vi "Read_VN200.vi"(0 "FPGA Interface":refnum<k20>, 5 "error in":errorcluster) -> (4 "FPGA Interface Out":refnum<k20>, 6 "error out":errorcluster, 8 "Position Data":T1)   [LabVIEW 2016]
uses:
  Typedef/INS Data.ctl
  <vilib>/Utility/error.llb/Error Cluster From Error Code.vi
  <vilib>/rvi/errors/niLvFpgaAdjustHostInterfaceError.vi
  <vilib>/rvi/interface/nirviReadWriteControl/nirviReadWriteControl.xnode
  NiFpgaLv.dll
  <vilib>/rvi/interface/Simulation/niFpgaSimulationCallBeginRW.vi
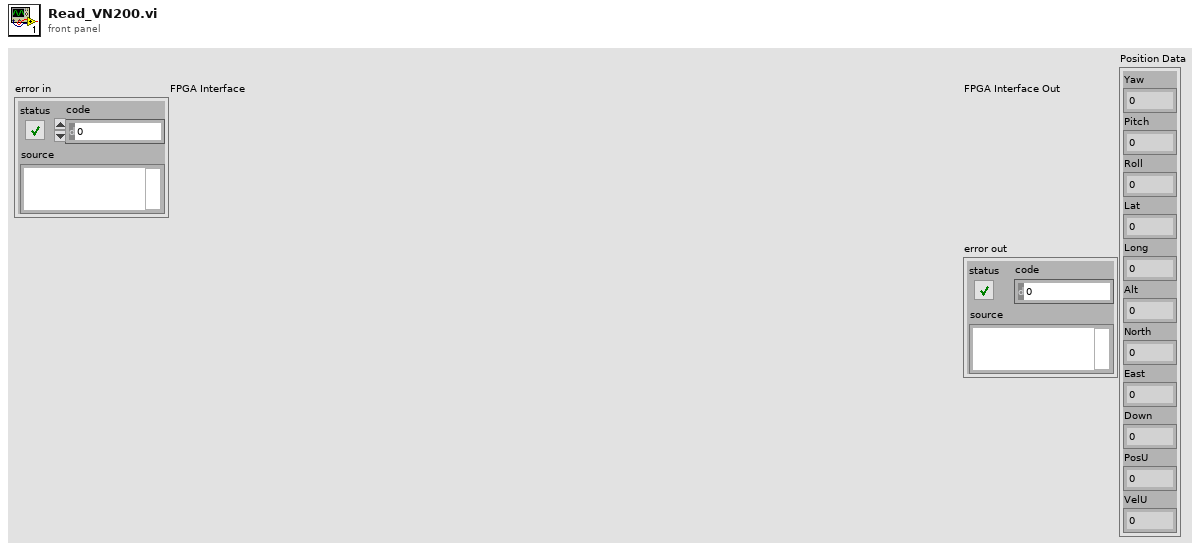
[diagram p1: front panel]
types:
  T1 = typedef "INS Data.ctl" = cluster{"Yaw":sgl, "Pitch":sgl, "Roll":sgl, "Lat":dbl, "Long":dbl, "Alt":dbl, "North":dbl, "East":dbl, "Down":dbl, "PosU":dbl, "VelU":dbl}
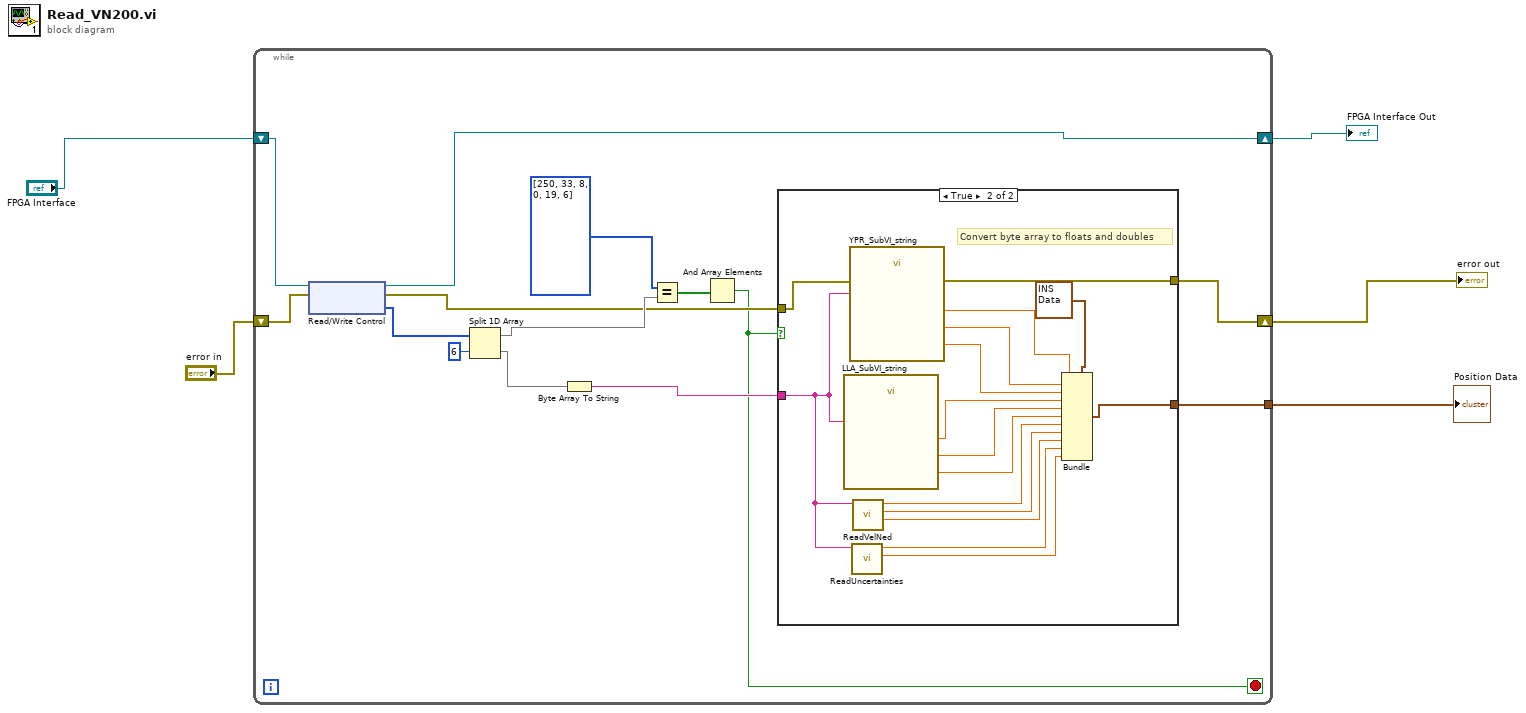
[diagram p0: block diagram]
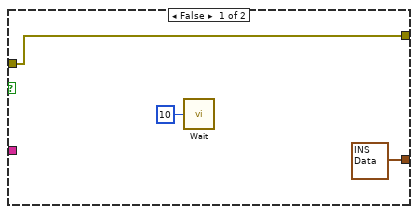
[diagram p2: hidden frame]
diagram:
  n1 = while {
    shift-right: [w10] -> w4
    shift-left: "error in" -> [w12]
    shift-right: [w9] -> w2
    shift-left: "FPGA Interface" -> [w8]
    tunnel: [w6] -> w1
    stop <- w7 stop-if-true
    n2 = xnode "Read/Write Control"("FPGA VI Reference In"=w8, "error in"=w12) -> ("FPGA VI Reference Out"=w9:refnum<k20>, "error out"=w11:errorcluster, "IMU_String"=w13:u8[])
    n3 = Split 1D Array(array=w13, index=6) -> (first subarray=w18:u8[], second subarray=w16:u8[])
    n4 = Byte Array To String(unsigned byte array=w16) -> (string=w17:string)
    n5 = Equal?(x=u8[] [250, 33, 8, 0, 19, 6] ("y"), y=w18) -> (x = y?=w19:bool[])
    n6 = And Array Elements(Boolean array=w19) -> (logical AND=w7:bool)
    n7 = case shown="True" w7 {
      tunnel: w17 -> [_ w27]
      tunnel: w11 -> [w22 w38]
      tunnel: [w22 w37] -> w10
      tunnel: [T1 {"Yaw"=0.0, "Pitch"=0.0, "Roll"=0.0, "Lat"=0.0, "Long"=0.0, "Alt"=0.0, "North"=0.0, "East"=0.0, "Down"=0.0, "PosU"=0.0, "VelU"=0.0} ("INS Data") w30] -> w6
      frame False {
        n8 = call "Wait"("Count(mSec)"=u32 10) -> ()  [unwired: 1 out]
      }
      frame True {
        # "Convert byte array to floats and doubles"
        n9 = call "LLA_SubVI_string.vi"("read buffer"=w27) -> ("Alt"=w31:dbl, "Long"=w32:dbl, "Lat"=w33:dbl)  [unwired: 8 in]
        n10 = call "YPR_SubVI_string.vi"("error in"=w38, "read buffer"=w27) -> ("error out"=w37:errorcluster, "Roll"=w34:sgl, "Pitch"=w35:sgl, "Yaw"=w36:sgl)  [unwired: 6 in]
        n11 = call "ReadUncertainties.vi"("read buffer"=w27) -> ("VelU"=w24:dbl, "PosU"=w25:dbl)  [unwired: 9 in]
        n12 = call "ReadVelNed.vi"("read buffer"=w27) -> ("Down"=w26:dbl, "East"=w28:dbl, "North"=w29:dbl)  [unwired: 8 in]
        n13 = Bundle(cluster=T1 {"Yaw"=0.0, "Pitch"=0.0, "Roll"=0.0, "Lat"=0.0, "Long"=0.0, "Alt"=0.0, "North"=0.0, "East"=0.0, "Down"=0.0, "PosU"=0.0, "VelU"=0.0} ("INS Data"), "Yaw"=w36, "Pitch"=w35, "Roll"=w34, "Lat"=w33, "Long"=w32, "Alt"=w31, "North"=w29, "East"=w28, "Down"=w26, "PosU"=w25, "VelU"=w24) -> (w30:T1)
      }
    }
  }
  "error out" <- w4
  "FPGA Interface Out" <- w2
  "Position Data" <- w1
